vi "Test Expression.vi"(10 "Cron Expression":string) -> ()   [LabVIEW 2013]
uses:
  Cron.Quartz/Cron.Quartz.lvclass
  Cron/Cron.lvclass/Cron.ctl
  Cron/Cron.lvclass
panel:
  out "Next Occurence (DST Corrected)":timestamp
  out "DST corrected":timestamp[](array[timestamp])
  out "Further occurences":timestamp[](array[timestamp])
  out "Next Occurence":timestamp
  in  "Update Cron Expression":string
  out "valid?":bool
  out "updated":bool
  out "Expression":string
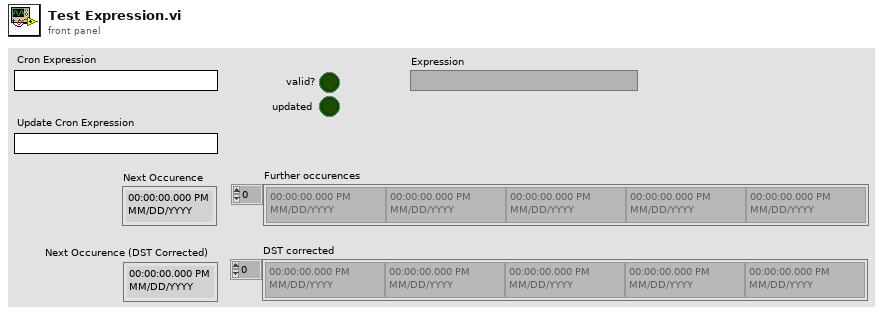
[diagram p1: front panel]
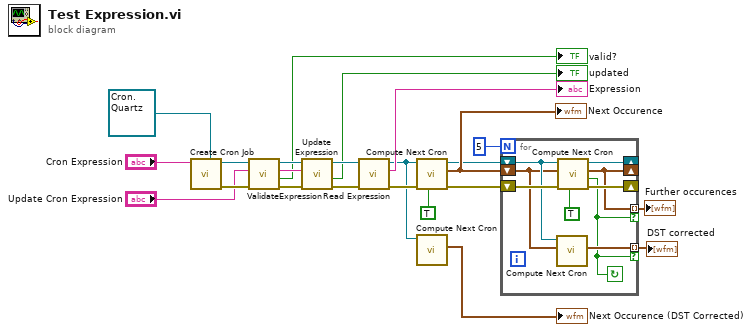
[diagram p0: block diagram]
diagram:
  n1 = call "Create Cron Job.vi"("Cron in"=refnum<class "Cron.Quartz.lvclass"> refnum ("openCron.lvlib:Cron.Quartz.lvclass"), "Cron Expression"="Cron Expression") -> ("error out"=w17:errorcluster, "Cron out"=w23:refnum<class "Cron.Quartz.lvclass">)  [unwired: 7 in, 1 out]
  n2 = call "ValidateExpression.vi"("error in (no error)"=w17, "Expression"="Update Cron Expression", "Cron in"=w23) -> ("error out"=w18:errorcluster, "valid?"=→"valid?":bool, "Expression dup"=w22:string, "Cron out"=w21:refnum<class "Cron.Quartz.lvclass">)  [unwired: 5 in]
  n3 = call "Update Expression.vi"("error in (no error)"=w18, "Expression"=w22, "Cron in"=w21) -> ("error out"=w19:errorcluster, "valid"=→"updated":bool, "Cron out"=w20:refnum<class "Cron.Quartz.lvclass">)  [unwired: 6 in]
  n4 = call "Read Expression.vi"("error in (no error)"=w19, "Cron in"=w20) -> ("error out"=w10:errorcluster, "Expression"=→"Expression":string, "Cron out"=w2:refnum<class "Cron.Quartz.lvclass">)  [unwired: 7 in]
  n5 = call "Compute Next Cron.vi"("Ignore DST?"=TRUE, "error in (no error)"=w10, "Cron in"=w2) -> ("error out"=w9:errorcluster, "Next Occurence"=w8:timestamp, "Cron out"=w6:refnum<class "Cron.Quartz.lvclass">)  [unwired: 5 in, 1 out]
  "Next Occurence" <- w8
  n6 = call "Compute Next Cron.vi"("Cron in"=w2) -> ("Next Occurence"=→"Next Occurence (DST Corrected)":timestamp)  [unwired: 7 in, 3 out]
  n7 = for {
    N: 5 -> [_]
    shift-right: [w31] -> _
    shift-left: w9 -> [w32]
    shift-right: [w30] -> _
    shift-left: w6 -> [w27]
    shift-right: [w28] -> _
    shift-left: w8 -> [w26]
    tunnel: [w28] -> w5 mode=indexing if=w24
    tunnel: [w25] -> w3 mode=indexing if=w24
    stop <- w24 continue-if-true
    n8 = call "Compute Next Cron.vi"("Time Stamp (Now)"=w26, "Cron in"=w27) -> ("Next Occurence"=w25:timestamp)  [unwired: 6 in, 3 out]
    n9 = call "Compute Next Cron.vi"("Ignore DST?"=TRUE, "error in (no error)"=w32, "Time Stamp (Now)"=w26, "Cron in"=w27) -> ("error out"=w31:errorcluster, "Occurence found"=w24:bool, "Next Occurence"=w28:timestamp, "Cron out"=w30:refnum<class "Cron.Quartz.lvclass">)  [unwired: 4 in]
  }
  "Further occurences" <- w5
  "DST corrected" <- w3
